vi "Change_Temp_Setpoint.vi"(2 "Debug Mode":bool, 3 "Elapsed Time (s)":dbl, 4 "State":enum16{"Edit", "Start", "Run", "End", "Idle"}(ring), 5 "Argument List In":string[](array[string])) -> (0 "Status Out":string, 1 "Argument List Out":string[](array[string]))   [LabVIEW 2011]
panel:
  in  "Cancel":bool
  in  "OK":bool
  in  "Setpoint (C)":dbl
  # "Change setpoint\nwithout waiting\nfor target to be\nreached."
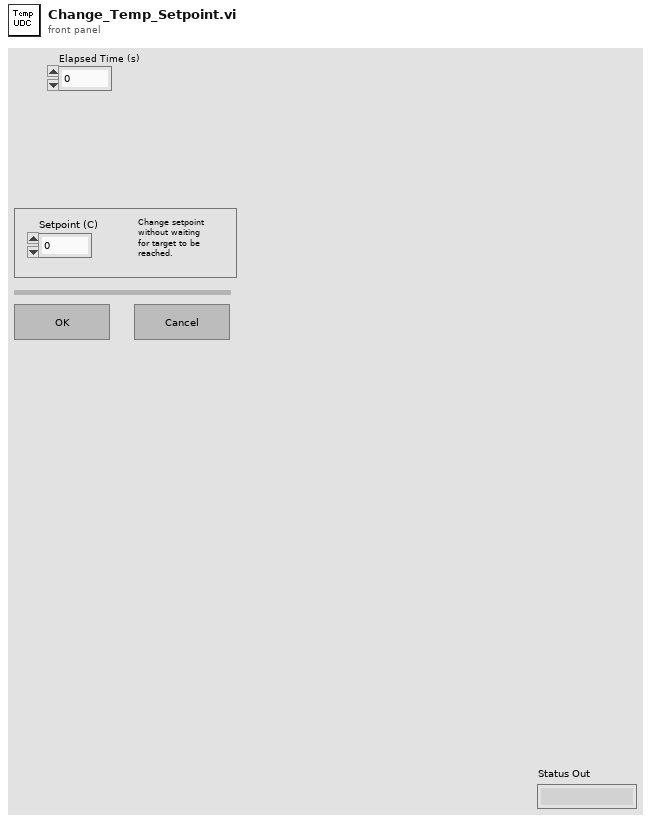
[diagram p1: front panel]
types:
  T1 = enum16{"Discrete", "Continuous", "Instantaneous"}
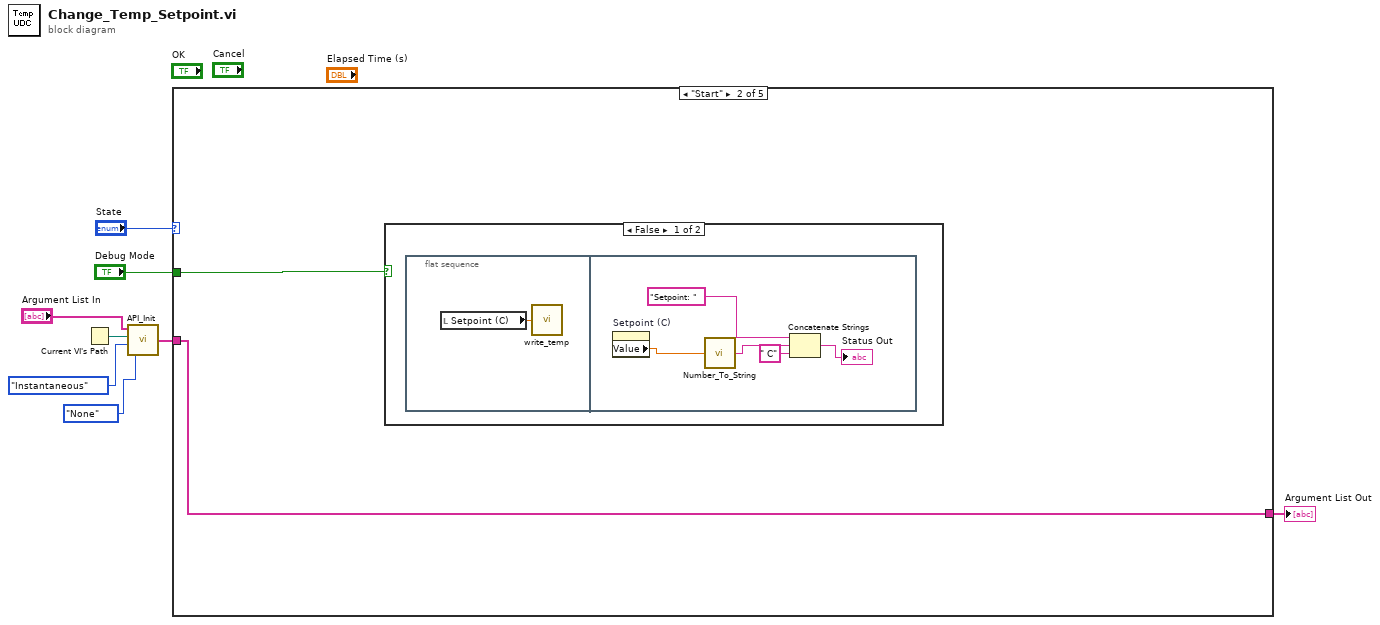
[diagram p0: block diagram]
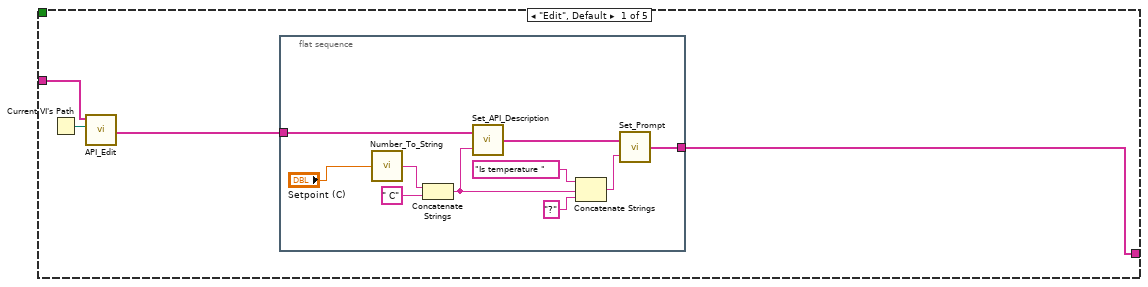
[diagram p2: hidden frame]
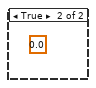
[diagram p3: hidden frame]
diagram:
  n1 = Current VI's Path() -> (path=w5:path)
  n2 = call "API_Init.vi"("API Option"=enum16{"None", "Blocking", "Wait for Input"}."None", "API Mode"=T1."Instantaneous", "VI Path"=w5, "Argument List In"="Argument List In") -> ("Argument List Out"=w2:string[])
  n3 = case shown="\"Start\"" "State" {
    tunnel: [w9 w24 w31 w32 w33] -> w7
    tunnel: w2 -> [w11 w24 w31 w32 w33]
    tunnel: "Debug Mode" -> [_ w23 _ _ _]
    frame "Edit", Default {
      n4 = Current VI's Path() -> (path=w12:path)
      n5 = call "API_Edit.vi"("VI Path"=w12, "Argument List In"=w11) -> ("Argument List Out"=w10:string[])  [unwired: 2 in]
      n6 = flat-sequence {
        tunnel: w10 -> [w16]
        tunnel: [w14] -> w9
        frame #0 {
          n7 = call "Number_To_String.vi"("Number"="Setpoint (C)") -> ("String"=w15:string)
          n8 = Concatenate Strings(w15, " C" ("string")) -> (w20:string)
          n9 = call "Set_API_Description.vi"("Description"=w20, "Argument List In"=w16) -> ("Argument List Out"=w21:string[])
          n10 = Concatenate Strings("Is temperature " ("Prompt"), w20, "?" ("string")) -> (w17:string)
          n11 = call "Set_Prompt.vi"("Prompt"=w17, "Argument List In"=w21) -> ("Argument List Out"=w14:string[])
        }
      }
    }
    frame "Start" {
      n12 = case shown="False" w23 {
        frame False {
          n13 = flat-sequence {
            frame #0 {
              n14 = local read "Setpoint (C)"() -> (w25:dbl)
              n15 = call "write_temp.vi"("Temperature (C)"=w25) -> ()  [unwired: 1 out]
            }
            frame #1 {
              n16 = property on="Setpoint (C)" class="DigNum (strict)"() -> ("Value"=w28:dbl)  [unwired: 2 in, 2 out]
              n17 = call "Number_To_String.vi"("Number"=w28) -> ("String"=w27:string)
              n18 = Concatenate Strings("Setpoint: " ("string"), w27, " C" ("string")) -> (→"Status Out":string)
            }
          }
        }
        frame True {
          (unwired) 0.0 ("Temperature (C)")
        }
      }
    }
    frame "Run" {
    }
    frame "End" {
    }
    frame "Idle" {
    }
  }
  "Argument List Out" <- w7
